vi "SVT THD+N.vi"   [LabVIEW 2017, in "SoundVib_Distortion.lvlib"]
doc: "Performs a total harmonic distortion plus noise (THD+N) analysis, including measuring the fundamental tone, and returns the detected fundamental frequency, detected fundamental amplitude, and THD+N. Signal in noise and distortion (SINAD) is the negative of THD+N in dB. Wire data to the<B> scaled signal [EU]</B> input to determine the polymorphic instance to use or manually select the instance.\n\nThe following formula calculates THD+N:\n\nTHD+N = sqrt(H^2 + N^2) / sqrt(F^2 + N^2 + H^2)\n\nwhere H is the harmonic RMS level, N is the noise RMS level, and F is the fundamental tone RMS level."
uses:
  <vilib>/addons/Sound and Vibration/svt_Distortion/SoundVib_Distortion.lvlib
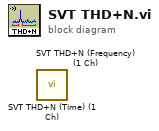
[diagram p0: block diagram]
diagram:
  n1 = call <vilib>:"SVT THD+N (Time) (1 Ch).vi"() -> ()  [unwired: 14 in, 6 out]
  n2 = call <vilib>:"SVT THD+N (Frequency) (1 Ch).vi"() -> ()  [unwired: 14 in, 6 out]
